vi "MAIN_save_embryos_positions.vi"(0 "Contrast image":T2, 1 "Image contrast":cluster{i32, i32}(slide)={16000, 0} scale=0.0..16000.0, 2 "XY REF cluster":T1, 3 "New Image":T2, 4 "queue ASI stage":refnum<queue>, 5 "ROI manager":refnum<vi>, 7 "ROI manager":i32(listbox), 9 "Start acquisition":bool, 11 "error in":errorcluster, 12 "XY positions":refnum<vi>, 13 "XY graph":cluster{dbl[], dbl[]}[](array[cluster])) -> (6 "XY REF cluster OUT":T1, 8 "Next task":T3, 14 "XY graph OUT":cluster{dbl[], dbl[]}[](array[cluster]), 15 "error out":errorcluster)   [LabVIEW 2015]
uses:
  CONTROLS/Q_main_element.ctl
  <vilib>/vision/Image Controls.llb/IMAQ Image.ctl
  CONTROLS/Q_ASI_stage_element.ctl
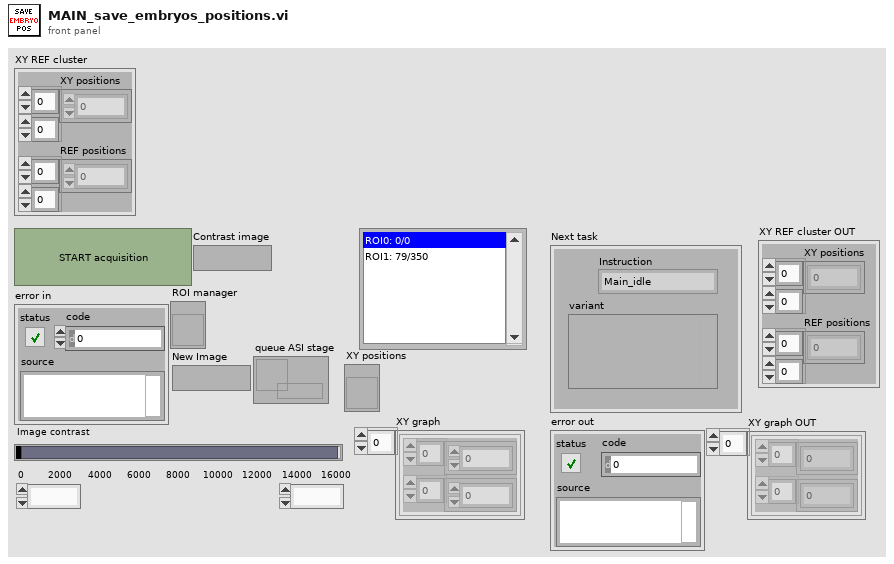
[diagram p1: front panel]
types:
  T1 = cluster{"XY positions":dbl[][], "REF positions":dbl[][]}
  T2 = typedef "IMAQ Image.ctl" = refnum<image>
  T3 = typedef "Q_main_element.ctl" = cluster{"variant":variant, "Instruction":enum16{"Main_idle", "Main_initialize", "Main_initialize_TDMS", "Main_initialize_Queue", "Main_error", "Main_DAQ_initialization_results", "Main_ASI_initialization_results", "Main_Piezo_initialization_results", "Main_Valve_initialization_results", "Main_Pump_initialization_results", "Main_CAMERA_initialization_results", "Main_FPGA_initialization_results", "Main_DAQ_error", "Main_ASI_error", "Main_Piezo_error", "Main_CAMERA_error", "Main_Valve_error", "Main_Pump_error", "Main_FPGA_error", "Main_start_acquiring", "Main_not_acquiring", "Main_acquiring", "Main_stop_acquiring", "Main_change_exposure", "Main_change_z_scan_parameters", "Main_define_ROI", "Main_define_mosaic", "Main_read_kinetic_time", "Main_cooler", "Main_read_temperature", "Main_save_XY", "Main_load_XY", "Main_discard_XY", "Main_move_to_XY", "Main_measure_QPD", "Main_autofocus_calibration", "Main_autofocus_initialization", "Main_autofocus_stop", "Main_save_PID", "Main_change_H_valve_position", "Main_two_way_valve", "Main_save_movie", "Main_init_single_scan", "Main_single_scan", "Main_stop_single_scan", "Main_merFISH_illumination_parameters", "Main_merFISH_buffer_probe_list", "Main_merFISH_injections_procedure", "Main_merFISH_save_setpoint", "Main_merFISH_DAPI_parameters", "Main_merFISH_Brightfield_parameters", "Main_merFISH_save_embryo_ROI", "Main_merFISH_init", "Main_merFISH_resume", "Main_merFISH_start_autofocus", "Main_merFISH_open_close_valve_merFISH", "Main_merFISH_open_close_valve_photobleaching", "Main_merFISH_hybridization", "Main_merFISH_move_to_ROI", "Main_merFISH_wait_stabilization", "Main_merFISH_move_to_REF", "Main_merFISH_scan", "Main_merFISH_photobleaching_injection", "Main_merFISH_photobleaching", "Main_merFISH_send_email", "Main_merFISH_close", "Main_STOP"}}
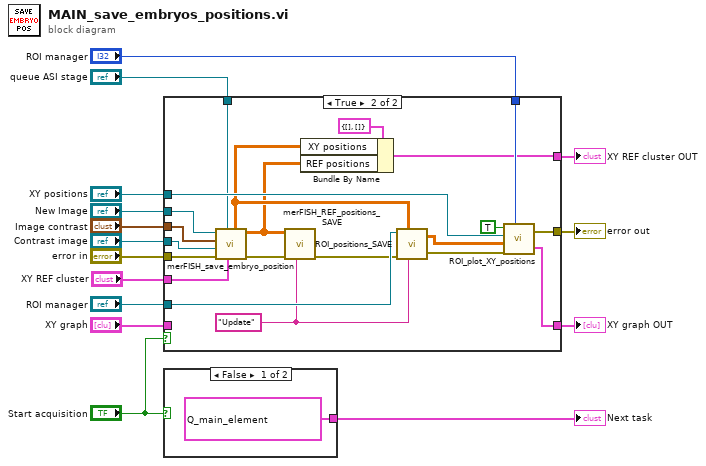
[diagram p0: block diagram]
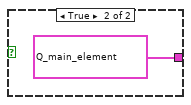
[diagram p2: hidden frame]
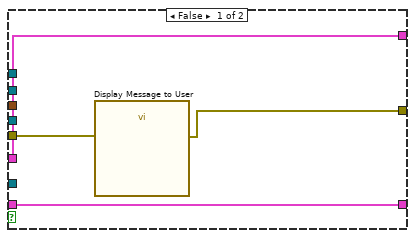
[diagram p3: hidden frame]
diagram:
  n1 = case shown="True" "Start acquisition" {
    tunnel: "Contrast image" -> [_ w40]
    tunnel: "error in" -> [w19 w39]
    tunnel: [w18 w34] -> w13
    tunnel: "XY REF cluster" -> [w16 w27]
    tunnel: "queue ASI stage" -> [_ w25]
    tunnel: "ROI manager" -> [_ w38]
    tunnel: "ROI manager" -> [_ w33]
    tunnel: "Image contrast" -> [_ w32]
    tunnel: "New Image" -> [_ w31]
    tunnel: "XY positions" -> [_ w30]
    tunnel: "XY graph" -> [w17 _]
    tunnel: [w17 w29] -> w3
    tunnel: [w16 w28] -> w1
    frame False {
      n2 = call "Display Message to User"("error in (no error)"=w19) -> ("error out"=w18:errorcluster)  [unwired: 9 in, 1 out]
    }
    frame True {
      w23 = "Update" ("Choice")
      n3 = call "merFISH_save_embryo_position.vi"("XY REF cluster"=w27, "queue ASI stage"=w25, "error in"=w39, "Image Dst"=w40, "Image contrast"=w32, "New Image"=w31) -> ("error out"=w24:errorcluster, "REF positions OUT"=w20:dbl[][], "XY positions OUT"=w21:dbl[][])  [unwired: 3 in]
      n4 = call "merFISH_REF_positions_SAVE.vi"("Choice"=w23, "error in"=w24, "REF positions"=w20) -> ("error out"=w22:errorcluster)  [unwired: 5 in, 1 out]
      n5 = Bundle By Name(cluster=T1 {"XY positions"=[], "REF positions"=[]} ("XY REF cluster"), "XY positions"=w21, "REF positions"=w20) -> (w28:T1)
      n6 = call "ROI_positions_SAVE.vi"("Choice"=w23, "XY positions"=w21, "error in"=w22, "ROI LstBox Refnum"=w38) -> ("error out"=w37:errorcluster, "XY positions OUT"=w36:dbl[][])  [unwired: 2 in]
      n7 = call "ROI_plot_XY_positions.vi"("Display?"=TRUE, "XYGraph Refnum"=w30, "XY positions"=w36, "error in"=w37, "ROI manager"=w33) -> ("error out"=w34:errorcluster, "XY graph"=w29:cluster{dbl[], dbl[]}[])
    }
  }
  "error out" <- w13
  "XY graph OUT" <- w3
  "XY REF cluster OUT" <- w1
  n8 = case shown="False" "Start acquisition" {
    tunnel: [T3 {"variant"=variant, "Instruction"=enum."Main_not_acquiring"} ("Q_main_element") T3 {"variant"=variant, "Instruction"=enum."Main_acquiring"} ("Q_main_element")] -> w14
    frame False {
    }
    frame True {
    }
  }
  "Next task" <- w14
